vi "Packet extractor.vi"(10 "Buffer in":string) -> (0 "Packets  read":string[](array[string]), 1 "N Packetes to read":i32, 3 "Buffer out":string)   [LabVIEW 2021]
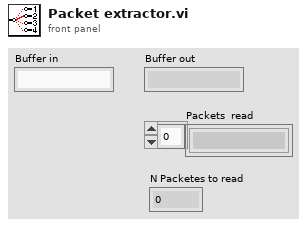
[diagram p1: front panel]
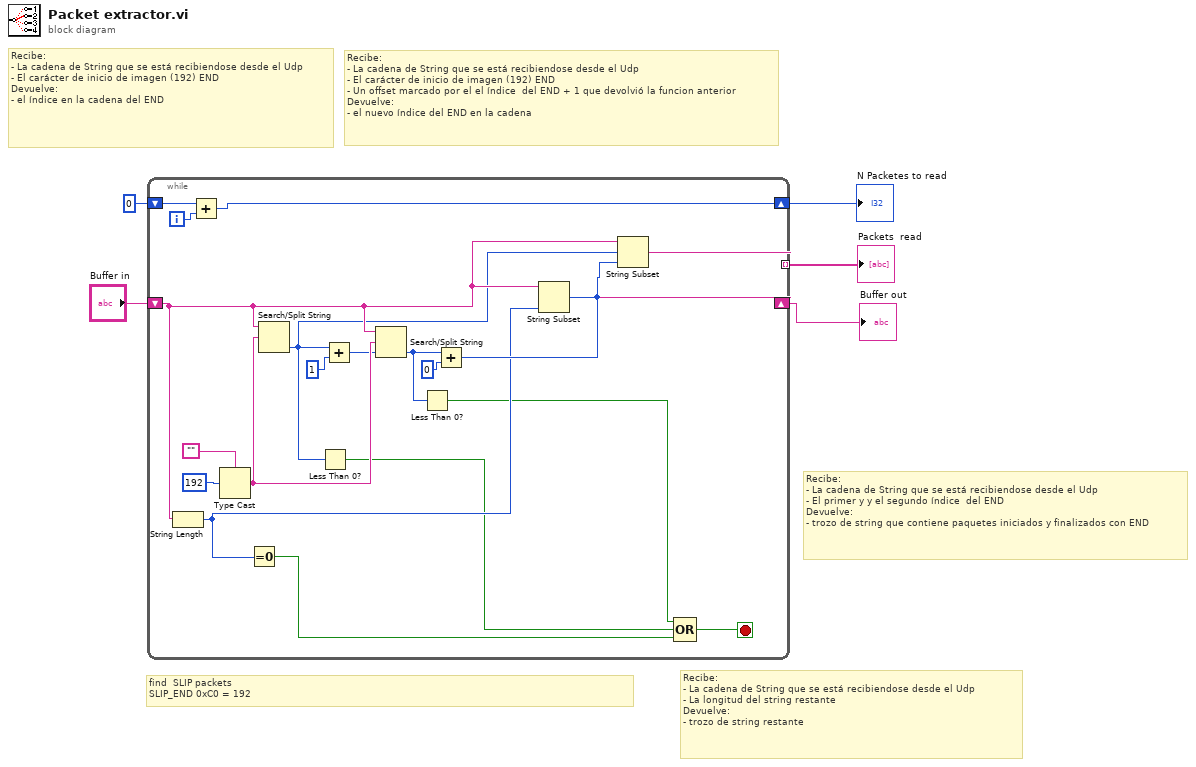
[diagram p0: block diagram]
diagram:
  # "Recibe:\n- La cadena de String que se está recibiendose desde el Udp\n- La longitud del string restante\nDevuelve:\n- trozo de string restante"
  # "Recibe:\n- La cadena de String que se está recibiendose desde el Udp\n- El primer y y el segundo índice  del END\nDevuelve:\n- trozo de string que contiene paquetes iniciados y finalizados con END"
  # "Recibe:\n- La cadena de String que se está recibiendose desde el Udp\n- El carácter de inicio de imagen (192) END\n- Un offset marcado por el el índice  del END + 1 que devolvió la funcion anterior \nDevuelve:\n- el nuevo índice del END en la cadena"
  # "Recibe:\n- La cadena de String que se está recibiendose desde el Udp\n- El carácter de inicio de imagen (192) END\nDevuelve:\n- el índice en la cadena del END"
  # "find  SLIP packets\nSLIP_END\t0xC0 = 192"
  n1 = while {
    shift-right: [w18] -> w1
    shift-left: "Buffer in" -> [w19]
    tunnel: [w13] -> w3 mode=indexing
    shift-right: [w14] -> w5
    shift-left: 0 -> [w15]
    i -> [w16]
    stop <- w11 stop-if-true
    n2 = String Length(string=w19) -> (length=w12:i32)
    n3 = Add(x=w15, y=w16) -> (x+y=w14:i32)
    n4 = Type Cast(type="", x=u8 192) -> (*(type *) &x=w23:string)
    n5 = Equal To 0?(x=w12) -> (x = 0?=w10:bool)
    n6 = Search/Split String(string=w19, search string/char (-)=w23) -> (offset of match=w17:i32)  [unwired: 1 in, 2 out]
    n7 = Less Than 0?(x=w17) -> (x < 0?=w8:bool)
    n8 = Add(x=w17, y=1) -> (x+y=w21:i32)
    n9 = Search/Split String(string=w19, search string/char (-)=w23, offset (0)=w21) -> (offset of match=w6:i32)  [unwired: 2 out]
    n10 = Less Than 0?(x=w6) -> (x < 0?=w9:bool)
    n11 = Add(x=w6, y=0 ("x")) -> (x+y=w20:i32)
    n12 = String Subset(string=w19, offset (0)=w20, length (rest)=w12) -> (substring=w18:string)
    n13 = String Subset(string=w19, offset (0)=w17, length (rest)=w20) -> (substring=w13:string)
    n14 = Compound Arithmetic op=OR(w9, w8, w10) -> (w11:bool)
  }
  "N Packetes to read" <- w5
  "Packets  read" <- w3
  "Buffer out" <- w1
